vi "GetDependencies.vi"(8 "error in (no error)":errorcluster, 11 "Enumerator in":u64[](array[numeric])) -> (0 "error out":errorcluster, 3 "Dependencies":T1[](array[typedef]) {"dependee"."component type" items=["standard", "hidden", "system", "unknown", "startup", "image", "essential"]; "depender"."component type" items=["standard", "hidden", "system", "unknown", "startup", "image", "essential"]})   [LabVIEW 2017, in "nisyscfg.lvlib"]
uses:
  <vilib>/nisyscfg/nisyscfg.lvlib
  <vilib>/nisyscfg/Broken Dependency 1.2.ctl
  <vilib>/nisyscfg/Software 1.2.ctl
  <vilib>/nisyscfg/Component Type.ctl
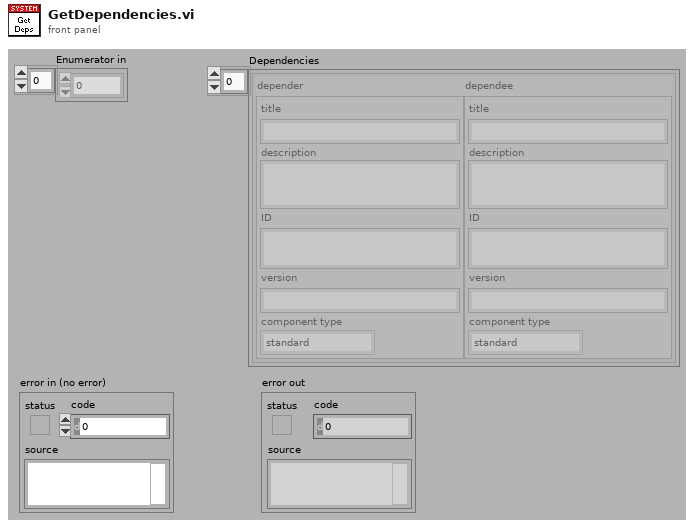
[diagram p1: front panel]
types:
  T1 = typedef "nisyscfg.lvlib/Broken Dependency 1.2.ctl" = cluster{"depender":T2, "dependee":T2}
  T2 = typedef "nisyscfg.lvlib/Software 1.2.ctl" = cluster{"title":string, "description":string, "ID":string, "version":string, "component type":T3}
  T3 = typedef "nisyscfg.lvlib/Component Type.ctl" = u32
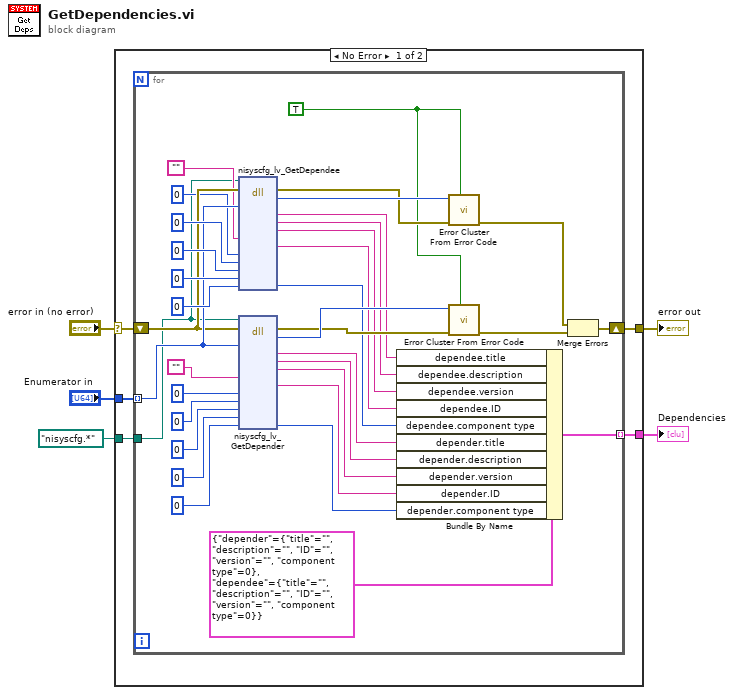
[diagram p0: block diagram]
diagram:
  n1 = case shown="No Error" "error in (no error)" {
    selector: "error in (no error)" -> [w7 w46]
    tunnel: [w10 w46] -> w5
    tunnel: "Enumerator in" -> [w9 _]
    tunnel: [w8 _] -> w3
    tunnel: path "nisyscfg.*" ("path in") -> [w6 _]
    frame No Error {
      n2 = for {
        tunnel: w9 -> [w33] mode=indexing
        shift-right: [w29] -> w10
        shift-left: w7 -> [w32]
        tunnel: [w26] -> w8 mode=indexing
        tunnel: w6 -> [w23]
        w11 = TRUE ("show call chain? (False)")
        n3 = dll-call lib="nisyscfg.*" fn="nisyscfg_lv_GetDependee" label="GetDependee"(path in=w23, error in=w32, "dependency"=w33, "oldestCompatibleVersion"="", "isAvailable"=u32 0, "hideVersion"=u32 0, "numChildren"=u32 0, "type"=u32 0, "visibilityType"=u32 0) -> (error out=w38:errorcluster, "result"=w39:i32, "title"=w21:string, "description"=w20:string, "version"=w19:string, "ID"=w18:string, "visibilityType"=w17:u32)  [unwired: 11 in, 1 out]
        n4 = dll-call lib="nisyscfg.*" fn="nisyscfg_lv_GetDepender" label="GetDepender"(path in=w23, error in=w32, "dependency"=w33, "oldestCompatibleVersion"="", "isAvailable"=u32 0, "hideVersion"=u32 0, "numChildren"=u32 0, "type"=u32 0, "visibilityType"=u32 0) -> (error out=w44:errorcluster, "result"=w45:i32, "title"=w12:string, "description"=w13:string, "version"=w14:string, "ID"=w15:string, "visibilityType"=w16:u32)  [unwired: 11 in, 1 out]
        n5 = Bundle By Name(cluster=T1 {"depender"={"title"="", "description"="", "ID"="", "version"="", "component type"=0}, "dependee"={"title"="", "description"="", "ID"="", "version"="", "component type"=0}} ("broken dependency"), "dependee.title"=w21, "dependee.description"=w20, "dependee.version"=w19, "dependee.ID"=w18, "dependee.component type"=w17, "depender.title"=w12, "depender.description"=w13, "depender.version"=w14, "depender.ID"=w15, "depender.component type"=w16) -> (w26:T1)
        n6 = call <vilib>:"Error Cluster From Error Code.vi"("show call chain? (False)"=w11, "error in (no error)"=w38, "error code (0)"=w39) -> ("error out"=w31:errorcluster)  [unwired: 6 in]
        n7 = call <vilib>:"Error Cluster From Error Code.vi"("show call chain? (False)"=w11, "error in (no error)"=w44, "error code (0)"=w45) -> ("error out"=w30:errorcluster)  [unwired: 6 in]
        n8 = Merge Errors(w31, w30) -> (w29:errorcluster)
      }
    }
    frame Error {
    }
  }
  "error out" <- w5
  "Dependencies" <- w3
